vi "Circular.vi"(5 "Direction":u16(ring) items=["Clockwise", "Counter-clockwise"], 6 "return immediately":bool, 7 "Speed":dbl, 8 "error in (no error)":errorcluster, 9 "XY End":dbl[](array[numeric]), 10 "XY Center":dbl[](array[numeric]), 11 "Gantry In":refnum<k24>) -> (0 "error IO":errorcluster, 3 "Gantry Out":refnum<k24>)   [LabVIEW 2018, in "Motion.lvclass"]
uses:
  Motion.lvclass
  C:/Program Files (x86)/Aerotech/A3200/LabVIEW/2010/Bin/Aerotech.A3200.dll
  Program Files (x86)/Aerotech/A3200/LabVIEW/2010/Bin/Aerotech.A3200.dll
  Drivers/Aerotech A3200/Motion/CircularCenter.vi
  Drivers/Aerotech A3200/Aerotech.lvlib
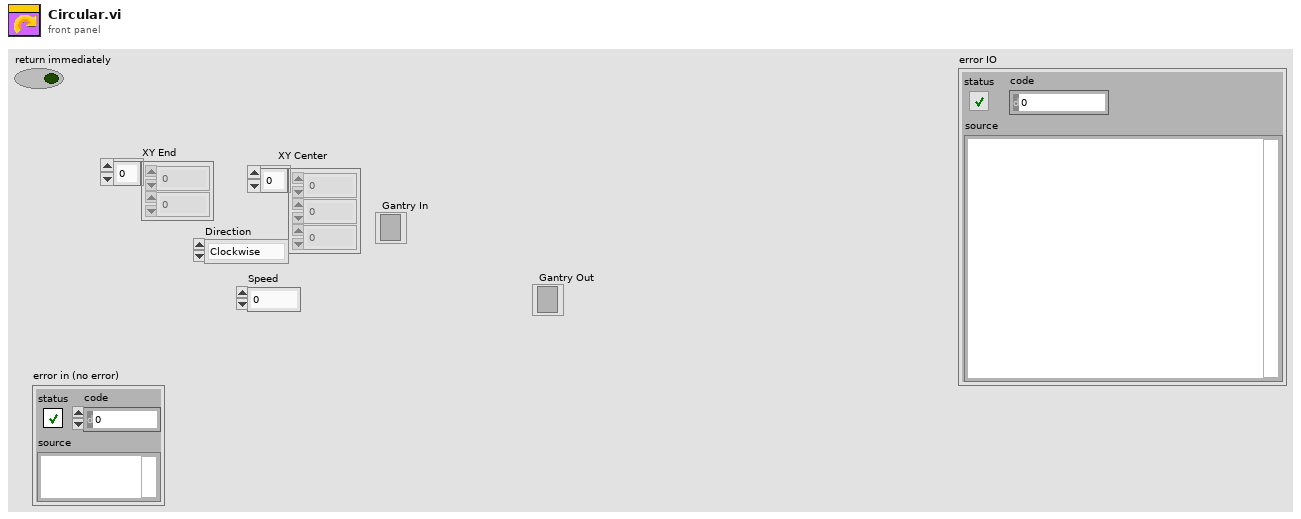
[diagram p1: front panel]
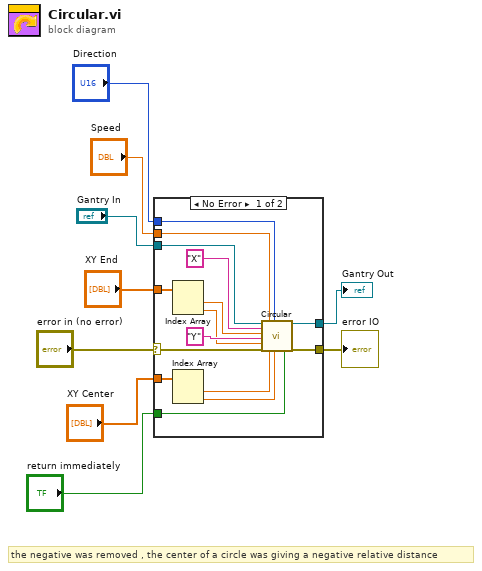
[diagram p0: block diagram]
diagram:
  # "the negative was removed , the center of a circle was giving a negative relative distance"
  n1 = case shown="No Error" "error in (no error)" {
    selector: "error in (no error)" -> [w19 w25]
    tunnel: "XY Center" -> [w23 _]
    tunnel: "Speed" -> [w18 _]
    tunnel: "Direction" -> [w24 _]
    tunnel: [w22 w26] -> w7
    tunnel: "Gantry In" -> [w21 w26]
    tunnel: [w20 w25] -> w5
    tunnel: "XY End" -> [w11 _]
    tunnel: "return immediately" -> [w10 _]
    frame No Error {
      n2 = Index Array(array=w11) -> (element #1=w16:dbl, element #2=w14:dbl)  [unwired: 2 in]
      n3 = Index Array(array=w23) -> (element #1=w13:dbl, element #2=w12:dbl)  [unwired: 2 in]
      n4 = call-poly "Circular.vi"("controller in"=w21, "axis 1 name"="X", "axis 1 endpoint"=w16, "axis 2 name"="Y", "axis 2 endpoint"=w14, "error in (no error)"=w19, "speed"=w18, "axis 1 center point"=w13, "direction"=w24, "axis 2 center point"=w12, "return immediately"=w10) -> ("controller out"=w22:refnum<k24>, "error out"=w20:errorcluster)  [unwired: 7 in]
    }
    frame Error {
    }
  }
  "Gantry Out" <- w7
  "error IO" <- w5
